vi "nominal_channel_writer.write_batches.path.vi"() -> (2 "Path":string="storage/writer/v1")   [LabVIEW 2020, in "Nominal Client.lvclass"]
uses:
  Nominal Client.lvclass
  Nominal Client.lvclass/Nominal Client.ctl
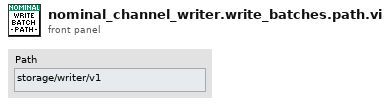
[diagram p1: front panel]
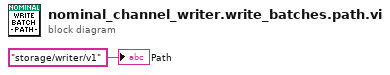
[diagram p0: block diagram]
diagram:
  "Path" <- "storage/writer/v1" ("Path")
